vi "Field_Step_gustav.vi"() -> ()   [LabVIEW 2019]
uses:
  Global/Global Variables/global.vi
  Instrument_Setup.vi
  Monitors/Utility/Monitor Communication/sub-vis/16T_Open_Queue.vi
  Global/Global Variables/Data_Display_global.vi
  Monitors/Utility/Monitor Communication/sub-vis/16T_Split_Cluster.vi
  Monitors/Utility/Monitor Communication/sub-vis/16T_Queue_Commands.vi
  Monitors/Utility/Monitor Communication/sub-vis/20T_Open_Queue.vi
  Monitors/Utility/Monitor Communication/sub-vis/20T_Split_Cluster.vi
  Monitors/Utility/Monitor Communication/sub-vis/20T_Queue_Commands.vi
panel:
  out "Array difference":dbl
  out "Lock-in Overload":bool[](array[boolean])
  out "Lock-in stable":bool
  out "Array min value":dbl
  out "Array max value":dbl
  out "Lock-in Values":dbl[](array[numeric])
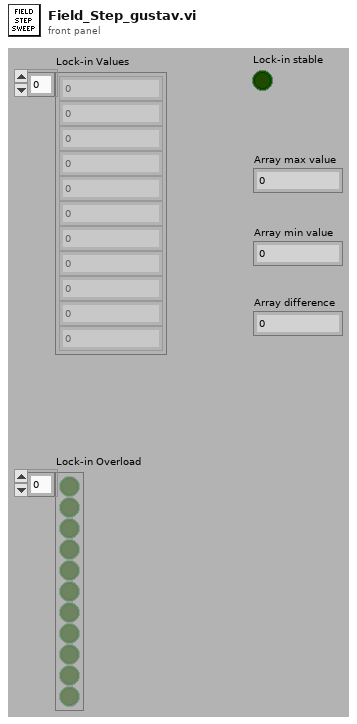
[diagram p1: front panel]
types:
  T1 = typedef "16T-Cluster.ctl" = cluster{"Clamp":bool, "Switch Heater":bool, "Go to Zero":bool, "Go to set":bool, "Go to Hold":bool, "Clamped":bool, "Quenched":bool, "Rate limit":bool, "Persistent":bool, "Hold":bool, "Set":bool, "Zero":bool, "Magnet (T)":dbl, "Leads (T)":dbl, "Magnet T (K)":dbl, "Switch":bool, "Setpoint (T)":dbl, "Rate (T/min)":dbl, "Select":bool, "Sweeping":bool}
  T2 = typedef "16T_Control.ctl" = cluster{"Clamp":bool, "Switch Heater":bool, "Go to Zero":bool, "Go to Set":bool, "Go to Hold":bool, "Setpoint (T)":dbl, "Rate (T/min)":dbl, "Set Rate":bool}
  T3 = typedef "15T-Cluster.ctl" = cluster{"Magnet (T)":dbl, "Leads (T)":dbl, "Setpoint (T)":dbl, "Rate (T/min)":dbl, "Set":bool, "Zero":bool, "Hold":bool, "Go to zero":bool, "Go to Hold":bool, "Go to Set":bool, "Clamp":bool, "Switch Heater":bool, "Rate limit":bool, "Switch":bool, "Clamped":bool, "Persistent":bool, "Quenched":bool, "Sweeping":bool, "Select":bool}
  T4 = typedef "15T-Control.ctl" = cluster{"Setpoint (T)":dbl, "Rate (T/min)":dbl, "Go to zero":bool, "Go to Hold":bool, "Go to Set":bool, "Clamp":bool, "Switch Heater":bool}
  T5 = typedef "20T_Cluster.ctl" = cluster{"Clamp":bool, "Switch Heater":bool, "Go to Zero":bool, "Go to set":bool, "Go to Hold":bool, "Clamped":bool, "Hold":bool, "Set":bool, "Zero":bool, "Magnet (T)":dbl, "Leads (T)":dbl, "Magnet T (K)":dbl, "Switch":bool, "Target Field (T)":dbl, "Field Setpoint (T)":dbl, "Rate Setpoint (T/min)":dbl, "Set Rate":bool, "Rate\n(T/min) ":dbl, "lambda NV (%)":dbl, "lambda p (mbar)":dbl, "lambda-Control":bool, "Activate lambda control":bool, "lambda NV  SP":dbl, "Set lambda NV":bool, "PSU Status":string, "PSU\nVoltage":dbl}
  T6 = typedef "20T_Status.ctl" = cluster{"Clamped":bool, "lambda-Control":bool, "Hold":bool, "Set":bool, "Zero":bool, "Magnet (T)":dbl, "Leads (T)":dbl, "Magnet T (K)":dbl, "Switch":bool, "Target Field (T)":dbl, "Rate (T/min)":dbl, "lambda NV (%)":dbl, "lambda p (mbar)":dbl, "PSU Status":string, "PSU Voltage":dbl}
  T7 = typedef "20T_Control.ctl" = cluster{"Clamp":bool, "Switch Heater":bool, "Go to Zero":bool, "Go to Set":bool, "Go to Hold":bool, "Field Setpoint (T)":dbl, "Rate Setpoint (T/min)":dbl, "Set Rate":bool, "Activate lambda control":bool, "Set lambda NV":bool, "lambda NV  SP":dbl}
  T8 = typedef "5T-Cluster.ctl" = cluster{"Go to set":bool, "Go to Zero":bool, "Clamp":bool, "Go to Hold":bool, "Clamped ":bool, "Quenched 2":bool, "Rate limit 2":bool, "Magnet (T)":dbl, "Leads (T)":dbl, "Rate (T/min)":dbl, "Sweeping":bool, "Setpoint":dbl, "Set":bool, "Zero":bool, "Hold":bool, "Clamp":bool}
  T9 = typedef "5T_Control.ctl" = cluster{"Rate (T/min)":dbl, "Setpoint":dbl, "Go to set":bool, "Go to Zero":bool, "Clamp":bool, "Go to Hold":bool, "Set Rate":bool}
  T10 = typedef "SR830-Cluster.ctl" = cluster{"Lockin 1":dbl[][], "X1-Display":dbl, "Y1-Display":dbl, "X1 Percent":dbl, "X1 Overload":bool, "Y1 Overload":bool, "Unit X1":string, "Unit X2":string, "Unit X2a":string, "Unit X1a":string, "Sensitivity Setpoint":i16, "X1 Percent 2":dbl, "Y1":dbl, "X1":dbl, "Preamp OVL":bool}
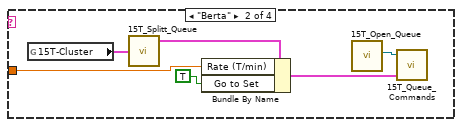
[diagram p2: hidden frame]
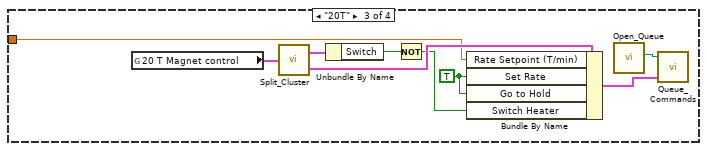
[diagram p3: hidden frame]
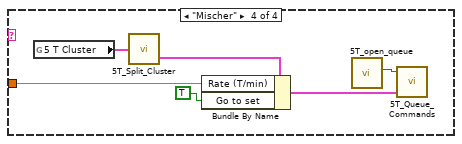
[diagram p4: hidden frame]
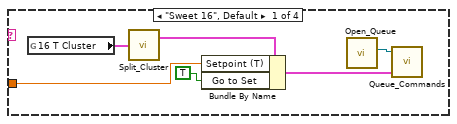
[diagram p5: hidden frame]
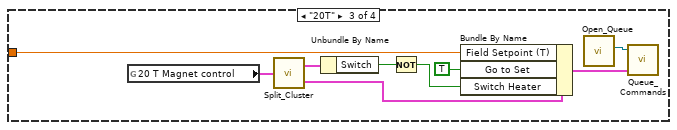
[diagram p6: hidden frame]
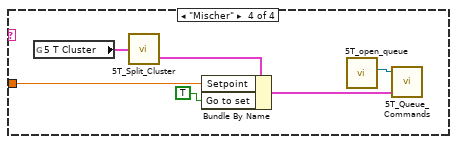
[diagram p7: hidden frame]
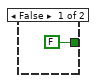
[diagram p9: hidden frame]
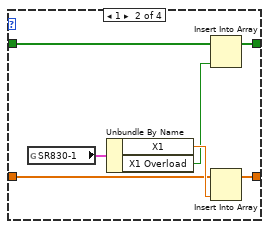
[diagram p13: hidden frame]
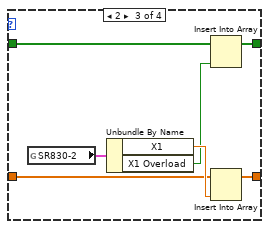
[diagram p14: hidden frame]
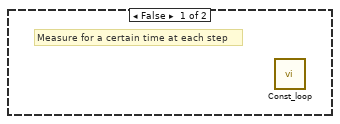
[diagram p15: hidden frame]
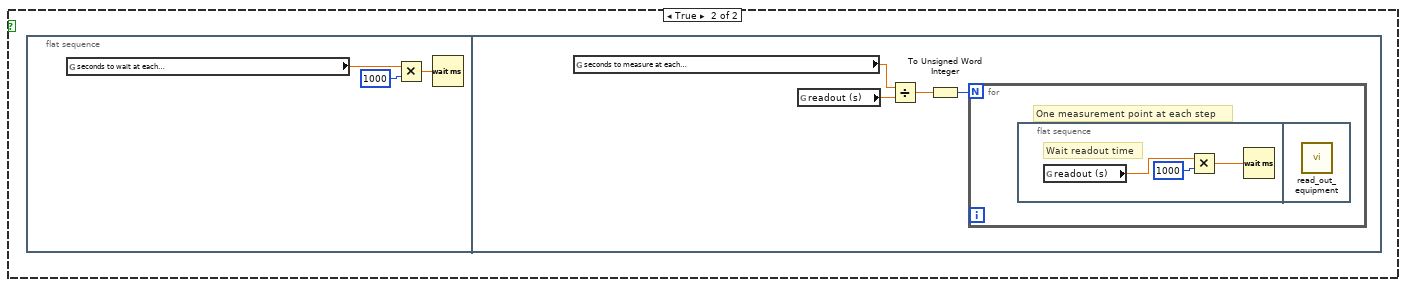
[diagram p16: hidden frame]
diagram:
  n1 = flat-sequence {
    frame #0 {
      n2 = global write "global.vi" "Cerrent State"(5) -> ()
    }
    frame #1 {
      n3 = global read "global.vi" "H Geschw.(T/min)"() -> (w2:dbl)
      n4 = global read "Instrument_Setup.vi" "Instrument"() -> (w3:string)
      n5 = case shown="\"Sweet 16\", Default" w3 {
        tunnel: w2 -> [w7 w10 w20 w25]
        frame "Sweet 16", Default {
          n6 = global read "Data_Display_global.vi" "16 T Cluster"() -> (w8:T1)
          n7 = call-poly "Split_Cluster.vi"("16 T Magnet control"=w8) -> ("16 T Magnet control"=w6:T2)  [unwired: 1 out]
          n8 = Bundle By Name(cluster=w6, "Rate (T/min)"=w7, "Go to Set"=TRUE) -> (w5:T2)
          n9 = call-poly "Open_Queue.vi"() -> ("queue out"=w9:refnum<queue>)  [unwired: 10 in, 1 out]
          n10 = call-poly "Queue_Commands.vi"("16 T Magnet control"=w5, "16T Queue"=w9) -> ()  [unwired: 1 in, 1 out]
        }
        frame "Berta" {
          n11 = global read "Data_Display_global.vi" "15T-Cluster"() -> (w14:T3)
          n12 = call "15T_Splitt_Queue.vi"("15T-Cluster"=w14) -> ("15T-Control"=w13:T4)  [unwired: 1 in, 1 out]
          n13 = Bundle By Name(cluster=w13, "Rate (T/min)"=w10, "Go to Set"=TRUE) -> (w11:T4)
          n14 = call "15T_Open_Queue.vi"() -> ("queue out"=w15:refnum<queue>)  [unwired: 10 in, 1 out]
          n15 = call "15T_Queue_Commands.vi"("15T-Control"=w11, "15T Queue"=w15) -> ()  [unwired: 1 in, 1 out]
        }
        frame "20T" {
          w16 = TRUE
          n16 = global read "Data_Display_global.vi" "20 T Magnet control"() -> (w23:T5)
          n17 = call-poly "Split_Cluster.vi"("20 T Cluster"=w23) -> ("20 T Status"=w19:T6, "20 T Control"=w21:T7)
          n18 = Unbundle By Name(w19) -> ("Switch"=w18:bool)
          n19 = Not(x=w18) -> (.not. x?=w17:bool)
          n20 = Bundle By Name(cluster=w21, "Rate Setpoint (T/min)"=w20, "Set Rate"=w16, "Go to Hold"=w16, "Switch Heater"=w17) -> (w22:T7)
          n21 = call-poly "Open_Queue.vi"() -> ("queue out"=w24:refnum<queue>)  [unwired: 10 in, 1 out]
          n22 = call-poly "Queue_Commands.vi"("20T Control (in)"=w22, "20T Queue"=w24) -> ()  [unwired: 1 in, 1 out]
        }
        frame "Mischer" {
          n23 = global read "Data_Display_global.vi" "5 T Cluster"() -> (w30:T8)
          n24 = call "5T_Split_Cluster.vi"("5 T Cluster"=w30) -> ("5T Control"=w29:T9)  [unwired: 1 out]
          n25 = Bundle By Name(cluster=w29, "Rate (T/min)"=w25, "Go to set"=TRUE) -> (w28:T9)
          n26 = call "5T_open_queue.vi"() -> ("queue out"=w27:refnum<queue>)  [unwired: 10 in, 1 out]
          n27 = call "5T_Queue_Commands.vi"("5T Control"=w28, "5T Queue"=w27) -> ()  [unwired: 1 in, 1 out]
        }
      }
    }
    frame #2 {
      # "2 seconds wait time for\nbetter communication\nwith Mercury iPS"
      n28 = Multiply(x=2, y=u32 1000 ("milliseconds to wait")) -> (x*y=w33:u32)
      n29 = Wait (ms)(milliseconds to wait=w33) -> ()  [unwired: 1 out]
    }
    frame #3 {
      n30 = while {
        i -> [w36]
        stop <- w35 stop-if-true
        n31 = flat-sequence {
          tunnel: [w37] -> w34
          tunnel: w36 -> [w45]
          tunnel: w34 -> [w50]
          tunnel: [w246] -> w35
          frame #0 {
            n32 = global read "global.vi" "number of steps in step sweep"() -> (w44:i32)
            n33 = global read "global.vi" "number of steps in step sweep"() -> (w42:i32)
            n34 = global read "global.vi" "H final (T)"() -> (w40:dbl)
            n35 = global read "global.vi" "H init.(T)"() -> (w39:dbl)
            n36 = Subtract(x=w40, y=w39) -> (x-y=w38:dbl)
            n37 = Subtract(x=w44, y=w45) -> (x-y=w41:i32)
            n38 = Subtract(x=w42, y=w41) -> (x-y=w43:i32)
            n39 = Divide(x=w38, y=w42) -> (x/y=w46:dbl)
            n40 = global read "global.vi" "H final (T)"() -> (w48:dbl)
            n41 = global write "Data_Display_global.vi" "current number of steps"(w43) -> ()
            n42 = Multiply(x=w41, y=w46) -> (x*y=w47:dbl)
            n43 = Subtract(x=w48, y=w47) -> (x-y=w37:dbl)
            n44 = global write "Data_Display_global.vi" "current field setpoint"(w37) -> ()
          }
          frame #1 {
            n45 = global read "Instrument_Setup.vi" "Instrument"() -> (w49:string)
            n46 = case shown="\"Berta\"" w49 {
              tunnel: w50 -> [w54 w57 w67 w72]
              frame "Sweet 16", Default {
                n47 = global read "Data_Display_global.vi" "16 T Cluster"() -> (w55:T1)
                n48 = call-poly "Split_Cluster.vi"("16 T Magnet control"=w55) -> ("16 T Magnet control"=w53:T2)  [unwired: 1 out]
                n49 = Bundle By Name(cluster=w53, "Setpoint (T)"=w54, "Go to Set"=TRUE) -> (w52:T2)
                n50 = call-poly "Open_Queue.vi"() -> ("queue out"=w56:refnum<queue>)  [unwired: 10 in, 1 out]
                n51 = call-poly "Queue_Commands.vi"("16 T Magnet control"=w52, "16T Queue"=w56) -> ()  [unwired: 1 in, 1 out]
              }
              frame "Berta" {
                n52 = global read "Data_Display_global.vi" "15T-Cluster"() -> (w61:T3)
                n53 = call "15T_Splitt_Queue.vi"("15T-Cluster"=w61) -> ("15T-Control"=w60:T4)  [unwired: 1 in, 1 out]
                n54 = Bundle By Name(cluster=w60, "Setpoint (T)"=w57, "Go to Set"=TRUE) -> (w58:T4)
                n55 = call "15T_Open_Queue.vi"() -> ("queue out"=w62:refnum<queue>)  [unwired: 10 in, 1 out]
                n56 = call "15T_Queue_Commands.vi"("15T-Control"=w58, "15T Queue"=w62) -> ()  [unwired: 1 in, 1 out]
              }
              frame "20T" {
                n57 = global read "Data_Display_global.vi" "20 T Magnet control"() -> (w70:T5)
                n58 = call-poly "Split_Cluster.vi"("20 T Cluster"=w70) -> ("20 T Status"=w66:T6, "20 T Control"=w68:T7)
                n59 = Unbundle By Name(w66) -> ("Switch"=w65:bool)
                n60 = Not(x=w65) -> (.not. x?=w64:bool)
                n61 = Bundle By Name(cluster=w68, "Field Setpoint (T)"=w67, "Go to Set"=TRUE, "Switch Heater"=w64) -> (w69:T7)
                n62 = call-poly "Open_Queue.vi"() -> ("queue out"=w71:refnum<queue>)  [unwired: 10 in, 1 out]
                n63 = call-poly "Queue_Commands.vi"("20T Control (in)"=w69, "20T Queue"=w71) -> ()  [unwired: 1 in, 1 out]
              }
              frame "Mischer" {
                n64 = global read "Data_Display_global.vi" "5 T Cluster"() -> (w77:T8)
                n65 = call "5T_Split_Cluster.vi"("5 T Cluster"=w77) -> ("5T Control"=w76:T9)  [unwired: 1 out]
                n66 = Bundle By Name(cluster=w76, "Setpoint"=w72, "Go to set"=TRUE) -> (w75:T9)
                n67 = call "5T_open_queue.vi"() -> ("queue out"=w74:refnum<queue>)  [unwired: 10 in, 1 out]
                n68 = call "5T_Queue_Commands.vi"("5T Control"=w75, "5T Queue"=w74) -> ()  [unwired: 1 in, 1 out]
              }
            }
          }
          frame #2 {
            # "Check if target field is reached"
            n69 = while {
              i -> [w78]
              stop <- w82 stop-if-true
              n70 = global read "Data_Display_global.vi" "current field setpoint"() -> (w86:dbl)
              n71 = flat-sequence {
                tunnel: w86 -> [w88]
                tunnel: [w88] -> w80
                tunnel: w80 -> [w89]
                tunnel: [w89] -> w79
                tunnel: w78 -> [w92]
                tunnel: [w124] -> w85
                tunnel: [w123] -> w84
                tunnel: [w122] -> w83
                tunnel: [w121] -> w81
                tunnel: w79 -> [w122]
                tunnel: w85 -> [w130]
                tunnel: w84 -> [w129]
                tunnel: w83 -> [w128]
                tunnel: [w127] -> w82
                tunnel: w81 -> [w126]
                frame #0 {
                  # "Wait 1 sec"
                  n72 = Wait (ms)(milliseconds to wait=1000) -> ()  [unwired: 1 out]
                }
                frame #1 {
                  # "Resend order to iPS if Field Setpoint is not reached after 10 mins"
                  n73 = Equal?(x=600, y=w92) -> (x = y?=w90:bool)
                  n74 = case shown="True" w90 {
                    tunnel: w89 -> [_ w94]
                    frame False {
                    }
                    frame True {
                      n75 = flat-sequence {
                        tunnel: w94 -> [w97]
                        tunnel: [w97] -> w93
                        tunnel: [w107] -> w95
                        tunnel: w93 -> [w107]
                        tunnel: [w113] -> w96
                        tunnel: w95 -> [w113]
                        tunnel: w96 -> [w115]
                        frame #0 {
                          n76 = Number To Engineering String(2:3, 4:w97) -> (0:w100:string)  [unwired: 2 in]
                          n77 = Concatenate Strings("Target Field of ", w100, " T in B Step not reached after 10 mins. Resending the command to the power supply.") -> (w102:string)
                          n78 = Bundle By Name(cluster=errorcluster {"status"=FALSE, "code"=0, "source"=""} ("error constant"), "code"=0, "status"=TRUE, "source"=w102) -> (w105:errorcluster)
                          n79 = call "Error_handler.vi"("error constant"=w105) -> ()
                        }
                        frame #1 {
                          n80 = global read "Data_Display_global.vi" "20 T Magnet control"() -> (w109:T5)
                          n81 = call-poly "Split_Cluster.vi"("20 T Cluster"=w109) -> ("20 T Control"=w111:T7)  [unwired: 1 out]
                          n82 = Bundle By Name(cluster=w111, "Go to Hold"=TRUE) -> (w110:T7)
                          n83 = call-poly "Open_Queue.vi"() -> ("queue out"=w112:refnum<queue>)  [unwired: 10 in, 1 out]
                          n84 = call-poly "Queue_Commands.vi"("20T Control (in)"=w110, "20T Queue"=w112) -> ()  [unwired: 1 in, 1 out]
                        }
                        frame #2 {
                          # "Wait 5 sec"
                          n85 = Wait (ms)(milliseconds to wait=5000) -> ()  [unwired: 1 out]
                        }
                        frame #3 {
                          n86 = global read "Data_Display_global.vi" "20 T Magnet control"() -> (w117:T5)
                          n87 = call-poly "Split_Cluster.vi"("20 T Cluster"=w117) -> ("20 T Control"=w119:T7)  [unwired: 1 out]
                          n88 = Bundle By Name(cluster=w119, "Go to Set"=TRUE, "Field Setpoint (T)"=w115) -> (w118:T7)
                          n89 = call-poly "Open_Queue.vi"() -> ("queue out"=w120:refnum<queue>)  [unwired: 10 in, 1 out]
                          n90 = call-poly "Queue_Commands.vi"("20T Control (in)"=w118, "20T Queue"=w120) -> ()  [unwired: 1 in, 1 out]
                        }
                      }
                    }
                  }
                }
                frame #2 {
                  n91 = global read "Instrument_Setup.vi" "Lower Limit\nSweep-Tolerance-\nMagnetic-Field (T)"() -> (w121:dbl)
                  n92 = global read "Instrument_Setup.vi" "Sweep-Tolerance-\nMagnetic-Field (%)"() -> (w123:dbl)
                  n93 = global read "Data_Display_global.vi" "Magnetic Field SC"() -> (w125:dbl)
                  n94 = call "H_check_2.vi"("Lower Limit\nSweep\nTolerance (T)"=w121, "Sweep\nTolerance %"=w123, "H_in"=w125, "H_target (K)"=w122) -> ("= H target"=w124:bool)  [unwired: 7 in]
                }
                frame #3 {
                  # "Check Stability every second for 5s"
                  n95 = case shown="True" w130 {
                    tunnel: w129 -> [_ w135]
                    tunnel: w128 -> [_ w134]
                    tunnel: [FALSE w133] -> w127
                    tunnel: w126 -> [_ w132]
                    frame False {
                    }
                    frame True {
                      n96 = while {
                        tunnel: w135 -> [w146]
                        tunnel: w134 -> [w144]
                        tunnel: [w138] -> w133
                        tunnel: w132 -> [w136]
                        i -> [w140]
                        stop <- w141 stop-if-true
                        n97 = flat-sequence {
                          tunnel: [w148] -> w145
                          tunnel: w144 -> [w148]
                          tunnel: [w147] -> w137
                          tunnel: w136 -> [w147]
                          tunnel: w146 -> [w154]
                          tunnel: w145 -> [w153]
                          tunnel: [w151] -> w143
                          tunnel: w137 -> [w150]
                          frame #0 {
                            # "Wait 1 sec"
                            n98 = Wait (ms)(milliseconds to wait=1000) -> ()  [unwired: 1 out]
                          }
                          frame #1 {
                            n99 = global read "Data_Display_global.vi" "Magnetic Field SC"() -> (w152:dbl)
                            n100 = call "H_check_2.vi"("Lower Limit\nSweep\nTolerance (T)"=w150, "Sweep\nTolerance %"=w154, "H_in"=w152, "H_target (K)"=w153) -> ("= H target"=w151:bool)  [unwired: 7 in]
                          }
                        }
                        n101 = Not(x=w143) -> (.not. x?=w142:bool)
                        n102 = Greater?(x=w140, y=5) -> (0:w138:bool)
                        n103 = Or(x=w142, y=w138) -> (x .or. y?=w141:bool)
                      }
                    }
                  }
                }
              }
            }
          }
          frame #3 {
            n104 = global read "Instrument_Setup.vi" "Measure for time of CC skript\nat each field step point"() -> (w157:bool)
            n105 = global read "global.vi" "-CC"() -> (w159:dbl)
            n106 = Not Equal?(x=w159, y=1) -> (x != y?=w156:bool)
            n107 = And(x=w157, y=w156) -> (x .and. y?=w155:bool)
            n108 = case shown="True" w155 {
              frame False {
              }
              frame True {
                n109 = call "create_data_file.vi"() -> ()  [unwired: 3 in]
              }
            }
          }
          frame #4 {
            # "Check if lock-in has a stable value for the specified amount of time"
            n110 = global read "Instrument_Setup.vi" "Wait until lock-in is\nsettled for each\nfield step point?"() -> (w160:bool)
            n111 = case shown="True" w160 {
              frame False {
              }
              frame True {
                n112 = global read "Instrument_Setup.vi" "seconds to check if lock-in\nis stable"() -> (w162:dbl)
                n113 = global read "Instrument_Setup.vi" "readout (s)"() -> (w163:dbl)
                n114 = Divide(x=w162, y=w163) -> (x/y=w164:dbl)
                n115 = To Unsigned Word Integer(number=w164) -> (unsigned 16bit integer=w161:u16)
                n116 = while {
                  tunnel: w161 -> [w166]
                  stop <- w167 stop-if-true
                  n117 = flat-sequence {
                    tunnel: [w174] -> w168
                    tunnel: w166 -> [w173]
                    tunnel: [w169] -> w165
                    tunnel: w168 -> [w222]
                    tunnel: [w215] -> w167
                    tunnel: w165 -> [w221]
                    frame #0 {
                      n118 = local write "Lock-in stable"(FALSE) -> ()
                      n119 = for {
                        N: w173 -> [_]
                        shift-right: [w180] -> w174
                        shift-left: dbl[] [] -> [w179]
                        shift-right: [w177] -> w169
                        shift-left: bool[] [] -> [w175]
                        n120 = flat-sequence {
                          tunnel: w179 -> [w185]
                          tunnel: [w185] -> w178
                          tunnel: [w181] -> w176
                          tunnel: w175 -> [w181]
                          tunnel: [w187] -> w180
                          tunnel: w178 -> [w189]
                          tunnel: [w186] -> w177
                          tunnel: w176 -> [w188]
                          frame #0 {
                            # "Wait readout time"
                            n121 = global read "Instrument_Setup.vi" "readout (s)"() -> (w184:dbl)
                            n122 = Multiply(x=w184, y=u32 1000 ("milliseconds to wait")) -> (x*y=w182:dbl)
                            n123 = Wait (ms)(milliseconds to wait=w182) -> ()  [unwired: 1 out]
                          }
                          frame #1 {
                            n124 = global read "Instrument_Setup.vi" "Which lock-in to check"() -> (w190:u16)
                            n125 = case shown="3" w190 {
                              tunnel: [w192 w196 w203 w210] -> w187
                              tunnel: w189 -> [w192 w197 w204 w211]
                              tunnel: [w191 w193 w200 w209] -> w186
                              tunnel: w188 -> [w191 w194 w202 w208]
                              frame 0, Default {
                              }
                              frame 1 {
                                n126 = global read "Data_Display_global.vi" "SR830-1"() -> (w199:T10)
                                n127 = Unbundle By Name(w199) -> ("X1"=w198:dbl, "X1 Overload"=w195:bool)
                                n128 = Insert Into Array(array=w194, new element=w195) -> (w193:bool[])  [unwired: 1 in]
                                n129 = Insert Into Array(array=w197, new element=w198) -> (w196:dbl[])  [unwired: 1 in]
                              }
                              frame 2 {
                                n130 = global read "Data_Display_global.vi" "SR830-2"() -> (w206:T10)
                                n131 = Unbundle By Name(w206) -> ("X1"=w205:dbl, "X1 Overload"=w201:bool)
                                n132 = Insert Into Array(array=w202, new element=w201) -> (w200:bool[])  [unwired: 1 in]
                                n133 = Insert Into Array(array=w204, new element=w205) -> (w203:dbl[])  [unwired: 1 in]
                              }
                              frame 3 {
                                n134 = global read "Data_Display_global.vi" "SR830-3"() -> (w213:T10)
                                n135 = Unbundle By Name(w213) -> ("X1"=w212:dbl, "X1 Overload"=w207:bool)
                                n136 = Insert Into Array(array=w208, new element=w207) -> (w209:bool[])  [unwired: 1 in]
                                n137 = Insert Into Array(array=w211, new element=w212) -> (w210:dbl[])  [unwired: 1 in]
                              }
                            }
                            "Lock-in Values" <- w187
                            "Lock-in Overload" <- w186
                          }
                        }
                      }
                    }
                    frame #1 {
                      n138 = Array Max & Min(array=w222) -> (max value=w225:dbl, min value=w224:dbl)  [unwired: 2 out]
                      "Array min value" <- w224
                      "Array max value" <- w225
                      n139 = Search 1D Array(1D array=w221, element=TRUE) -> (index of element=w219:i32)  [unwired: 1 in]
                      n140 = Subtract(x=w225, y=w224) -> (x-y=w214:dbl)
                      "Array difference" <- w214
                      n141 = global read "Instrument_Setup.vi" "Lock-in stability tolerance band (V)"() -> (w223:dbl)
                      n142 = Equal?(x=w219, y=-1) -> (x = y?=w216:bool)
                      n143 = Less?(x=w214, y=w223) -> (x < y?=w217:bool)
                      n144 = And(x=w216, y=w217) -> (x .and. y?=w215:bool)
                      "Lock-in stable" <- w215
                    }
                  }
                }
              }
            }
          }
          frame #5 {
            n145 = global read "Instrument_Setup.vi" "Take multiple data\npoints at each\nfield step point?"() -> (w226:bool)
            n146 = case shown="False" w226 {
              frame False {
                n147 = global read "Instrument_Setup.vi" "Measure for time of CC skript\nat each field step point"() -> (w228:bool)
                n148 = Not(x=w228) -> (.not. x?=w227:bool)
                n149 = case shown="True" w227 {
                  frame False {
                    # "Measure for a certain time at each step"
                    n150 = call "Const_loop.vi"() -> ()  [unwired: 4 in]
                  }
                  frame True {
                    # "One measurement point at each step"
                    n151 = flat-sequence {
                      frame #0 {
                        n152 = global read "Instrument_Setup.vi" "seconds to wait at each\nfield step in a step sweep"() -> (w231:dbl)
                        n153 = Multiply(x=w231, y=u32 1000 ("milliseconds to wait")) -> (x*y=w229:dbl)
                        n154 = Wait (ms)(milliseconds to wait=w229) -> ()  [unwired: 1 out]
                      }
                      frame #1 {
                        n155 = call "read_out_equipment.vi"() -> ()  [unwired: 1 in]
                      }
                    }
                  }
                }
              }
              frame True {
                n156 = flat-sequence {
                  frame #0 {
                    n157 = global read "Instrument_Setup.vi" "seconds to wait at each\nfield step in a step sweep"() -> (w234:dbl)
                    n158 = Multiply(x=w234, y=u32 1000 ("milliseconds to wait")) -> (x*y=w232:dbl)
                    n159 = Wait (ms)(milliseconds to wait=w232) -> ()  [unwired: 1 out]
                  }
                  frame #1 {
                    n160 = global read "Instrument_Setup.vi" "seconds to measure at each\nfield step in a step sweep"() -> (w238:dbl)
                    n161 = global read "Instrument_Setup.vi" "readout (s)"() -> (w237:dbl)
                    n162 = Divide(x=w238, y=w237) -> (x/y=w236:dbl)
                    n163 = To Unsigned Word Integer(number=w236) -> (unsigned 16bit integer=w235:u16)
                    n164 = for {
                      N: w235 -> [_]
                      # "One measurement point at each step"
                      n165 = flat-sequence {
                        frame #0 {
                          # "Wait readout time"
                          n166 = global read "Instrument_Setup.vi" "readout (s)"() -> (w241:dbl)
                          n167 = Multiply(x=w241, y=u32 1000 ("milliseconds to wait")) -> (x*y=w239:dbl)
                          n168 = Wait (ms)(milliseconds to wait=w239) -> ()  [unwired: 1 out]
                        }
                        frame #1 {
                          n169 = call "read_out_equipment.vi"() -> ()  [unwired: 1 in]
                        }
                      }
                    }
                  }
                }
              }
            }
          }
          frame #6 {
            n170 = global read "global.vi" "-CC"() -> (w244:dbl)
            n171 = global read "Data_Display_global.vi" "current field setpoint"() -> (w245:dbl)
            n172 = Add(x=w244, y=1) -> (x+y=w242:dbl)
            n173 = global write "global.vi" "-CC"(w242) -> ()
            n174 = global read "global.vi" "H final (T)"() -> (w247:dbl)
            n175 = Equal?(x=w247, y=w245) -> (x = y?=w246:bool)
          }
        }
      }
    }
  }
